vi "Logger.vi"() -> ()   [LabVIEW 2019]
panel:
  out "path":path
  out "error out":errorcluster
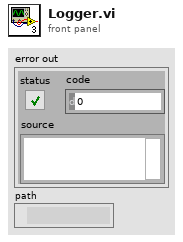
[diagram p1: front panel]
types:
  T1 = cluster{"ID":u8, "Command":sgl, "Error":sgl, "Status":u32, "TimeOutCnt":u32, "TimeOut":bool}
  T2 = enum16{"open", "replace", "create", "open or create", "replace or create", "replace or create with confirmation"}
  T3 = cluster{"ID":u8, "Command":sgl, "Error":sgl, "Status":u32, "TimeOutCnt":u32, "TimeOut":bool}[][][]
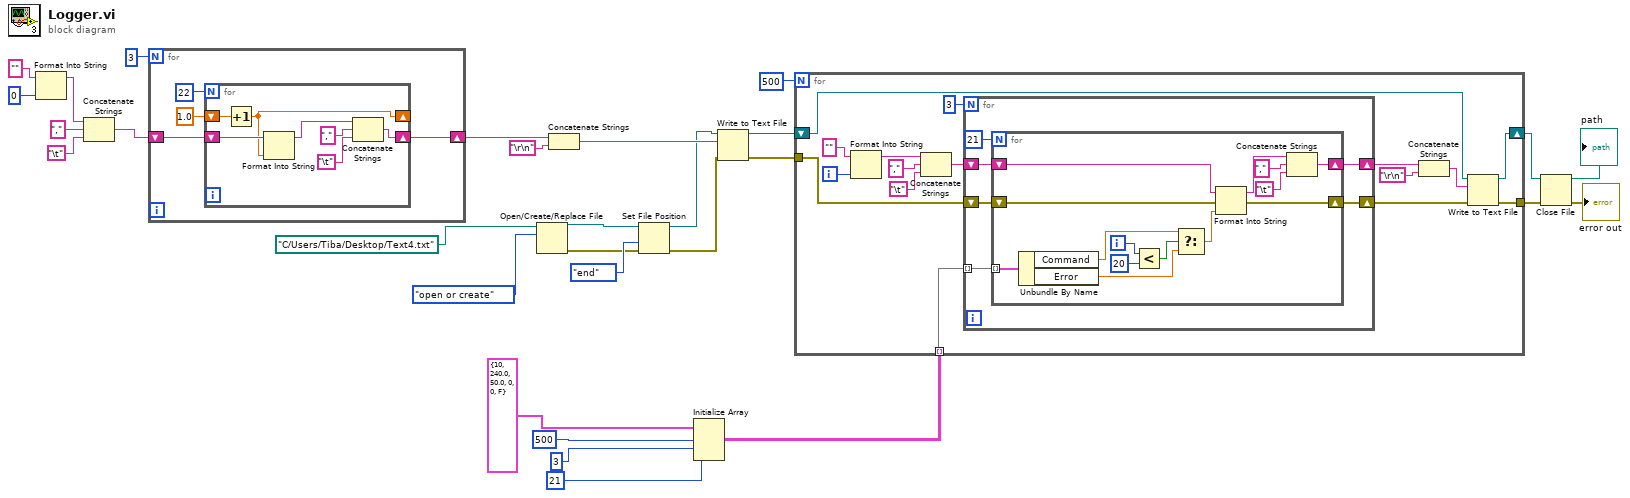
[diagram p0: block diagram]
diagram:
  n1 = Format Into String(initial string="", 0 ("input 1")) -> (resulting string=w26:string)  [unwired: 2 in, 1 out]
  n2 = Concatenate Strings(w26, ",", "\t") -> (w25:string)
  n3 = for {
    N: 3 -> [_]
    shift-right: [w31] -> w21
    shift-left: w25 -> [w32]
    n4 = for {
      N: 22 -> [_]
      shift-right: [w37] -> w31
      shift-left: w32 -> [w40]
      shift-right: [w35] -> _
      shift-left: 1.0 -> [w36]
      n5 = Increment(x=w36) -> (x+1=w35:dbl)
      n6 = Format Into String(initial string=w40, w35) -> (resulting string=w39:string)  [unwired: 2 in, 1 out]
      n7 = Concatenate Strings(w39, ",", "\t") -> (w37:string)
    }
  }
  n8 = Open/Create/Replace File(file path (use dialog)=path "C:/Users/Tiba/Desktop/Text4.txt", operation (0:open)=T2."open or create") -> (refnum out=w4:refnum<file>, error out=w1:errorcluster)  [unwired: 4 in, 1 out]
  n9 = Concatenate Strings(w21, "\r\n") -> (w20:string)
  n10 = Set File Position(refnum=w4, from (0:start)=enum16{"start", "end", "current"}."end" ("à partir de (0 : start)"), error in=w1) -> (refnum out=w3:refnum<file>, error out=w2:errorcluster)  [unwired: 1 in]
  n11 = Initialize Array(T1 {"ID"=10, "Command"=240.0, "Error"=50.0, "Status"=0, "TimeOutCnt"=0, "TimeOut"=FALSE} ("Sync"), 500 ("dimension size"), 3 ("dimension size"), 21 ("dimension size")) -> (w7:T3)
  n12 = Write to Text File(file (use dialog)=w3, text=w20, error in=w2) -> (refnum out=w17:refnum<file>, error out=w15:errorcluster)  [unwired: 1 in, 1 out]
  n13 = for {
    N: 500 -> [_]
    tunnel: w15 -> [w52]
    tunnel: [w50] -> w14
    shift-right: [w43] -> w12
    shift-left: w17 -> [w53]
    tunnel: w7 -> [w42] mode=indexing
    i -> [w49]
    n14 = Format Into String(initial string="", w49) -> (resulting string=w45:string)  [unwired: 2 in, 1 out]
    n15 = Concatenate Strings(w45, ",", "\t") -> (w44:string)
    n16 = for {
      N: 3 -> [_]
      tunnel: w42 -> [w62] mode=indexing
      shift-right: [w61] -> w55
      shift-left: w44 -> [w60]
      shift-right: [w59] -> w51
      shift-left: w52 -> [w58]
      n17 = for {
        N: 21 -> [_]
        tunnel: w62 -> [w76] mode=indexing
        shift-right: [w66] -> w61
        shift-left: w60 -> [w65]
        shift-right: [w64] -> w59
        shift-left: w58 -> [w63]
        i -> [w75]
        n18 = Unbundle By Name(w76) -> ("Command"=w69:sgl, "Error"=w68:sgl)
        n19 = Less?(x=w75, y=20) -> (x < y?=w70:bool)
        n20 = Select(t=w69, s=w70, f=w68) -> (s? t:f=w67:sgl)
        n21 = Format Into String(initial string=w65, error in=w63, w67) -> (resulting string=w73:string, error out=w64:errorcluster)  [unwired: 1 in]
        n22 = Concatenate Strings(w73, ",", "\t") -> (w66:string)
      }
    }
    n23 = Concatenate Strings(w55, "\r\n") -> (w54:string)
    n24 = Write to Text File(file (use dialog)=w53, text=w54, error in=w51) -> (refnum out=w43:refnum<file>, error out=w50:errorcluster)  [unwired: 1 in, 1 out]
  }
  n25 = Close File(refnum=w12, error in=w14) -> (path=→"path":path, error out=→"error out":errorcluster)
